vi "simulate-dashboard.vi"() -> ()   [LabVIEW 2019]
uses:
  <vilib>/Rock Robotics/WPI/ThirdParty/JAS_Junk/TrajLib/TypeDef/SWERVE_DRIVE_MODULE_POSITION.ctl
  <vilib>/Rock Robotics/WPI/ThirdParty/JAS_Junk/TrajLib/TypeDef/ROTATION2D.ctl
  <vilib>/Rock Robotics/WPI/ThirdParty/JAS_Junk/TrajLib/TypeDef/SWERVE_DRIVE_MODULE_STATE.ctl
  <vilib>/Rock Robotics/WPI/ThirdParty/JAS_Junk/TrajLib/TypeDef/CHASSIS_SPEEDS.ctl
  Swerve_Drive_System/SWERVE_DRIVE_GLOBALS.vi
  Simulation/SIMULATION_SIM_Globals.vi
  Sweve_Trajectory_Following/SWERVE_TRAJECTORY_GLOBALS.vi
  <vilib>/Rock Robotics/WPI/ThirdParty/JAS_Junk/TrajLib/Trajectory_Library.lvlib
panel:
  in  "Tab Control":T1(tab)
  out "Battery Voltage":dbl(graph)
  out "Swerve Motor Demands":T2(graph)
  out "Drive Motor Demands":T2(graph)
  out "Swerve Module Devices":T3(array[cluster])
  out "GyroReading_Degreees":dbl
  out "Encoder Distances":dbl[](array[numeric]) format="%17.2f"
  out "Encoder Velocities":dbl[](array[numeric]) format="%17.2f"
  out "Motor Demands":dbl[](array[numeric]) format="%17.2f"
  out "Battery Volts":dbl format="%16.2f"
  out "Swerve Module Positions":T4[](array[typedef]) {"Angle"."SIN" format="%13.4f"; "Angle"."COS" format="%13.4f"; "Angle"."VALUE" format="%13.4f"; "Distance" format="%19.2f"}
  out "Swerve Module States":T6[](array[typedef]) {"Angle"."SIN" format="%13.4f"; "Angle"."COS" format="%13.4f"; "Angle"."VALUE" format="%13.4f"; "Speed" format="%18.2f"}
  out "Adjusted Module State Demands":T6[](array[typedef]) {"Angle"."SIN" format="%13.4f"; "Angle"."COS" format="%13.4f"; "Angle"."VALUE" format="%13.4f"; "Speed" format="%20.2f"}
  out "Orientation Angle Dmd_Rad":dbl format="%17.3f"
  out "Drv Chassis Velocity DmD":T7 {"vOmega" format="%10.3f"; "vY" format="%10.3f"; "vX" format="%10.3f"}
  out "GyroHeading_Radians":dbl format="%17.2f"
  out "Orientation Angle Error_Rad":dbl format="%17.3f"
  out "Orientation Correct CO":dbl format="%17.3f"
  out "Adjusted Chassis Dmd":T7 {"vOmega" format="%10.3f"; "vY" format="%10.3f"; "vX" format="%10.3f"}
  out "Swerve Chassis Speed":T7 {"vOmega" format="%10.3f"; "vY" format="%10.3f"; "vX" format="%10.3f"}
  out "Mod Swerve in Deadband":bool
  out "Traj_OnTarget":bool
  # "SIMULATION"
  # "SWERVE DRIVE"
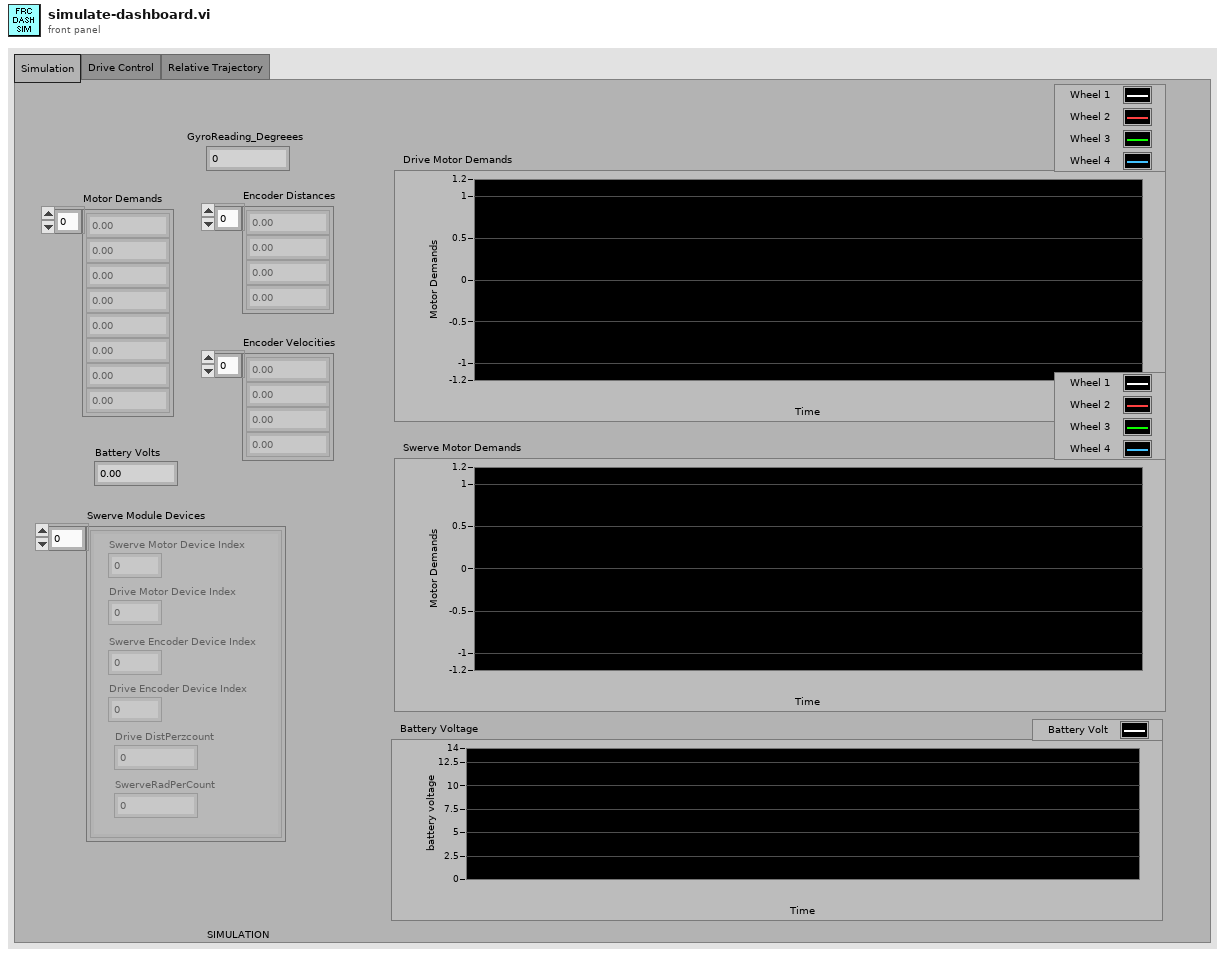
[diagram p1: front panel]
types:
  T1 = enum32{"Simulation", "Drive Control", "Relative Trajectory"}
  T2 = cluster{"Motor Dmd":dbl, "Motor Dmd":dbl, "Motor Dmd":dbl, "Motor Dmd":dbl}
  T3 = cluster{"Swerve Motor Device Index":i32, "Drive Motor Device Index":i32, "Swerve Encoder Device Index":i32, "Drive Encoder Device Index":i32, "Drive DistPerzcount":dbl, "SwerveRadPerCount":dbl}[]
  T4 = typedef "Trajectory_Library.lvlib/SWERVE_DRIVE_MODULE_POSITION.ctl" = cluster{"Distance":dbl, "Angle":T5, "P":bool}
  T5 = typedef "Trajectory_Library.lvlib/ROTATION2D.ctl" = cluster{"VALUE":dbl, "COS":dbl, "SIN":dbl}
  T6 = typedef "Trajectory_Library.lvlib/SWERVE_DRIVE_MODULE_STATE.ctl" = cluster{"Speed":dbl, "Angle":T5}
  T7 = typedef "Trajectory_Library.lvlib/CHASSIS_SPEEDS.ctl" = cluster{"vX":dbl, "vY":dbl, "vOmega":dbl}
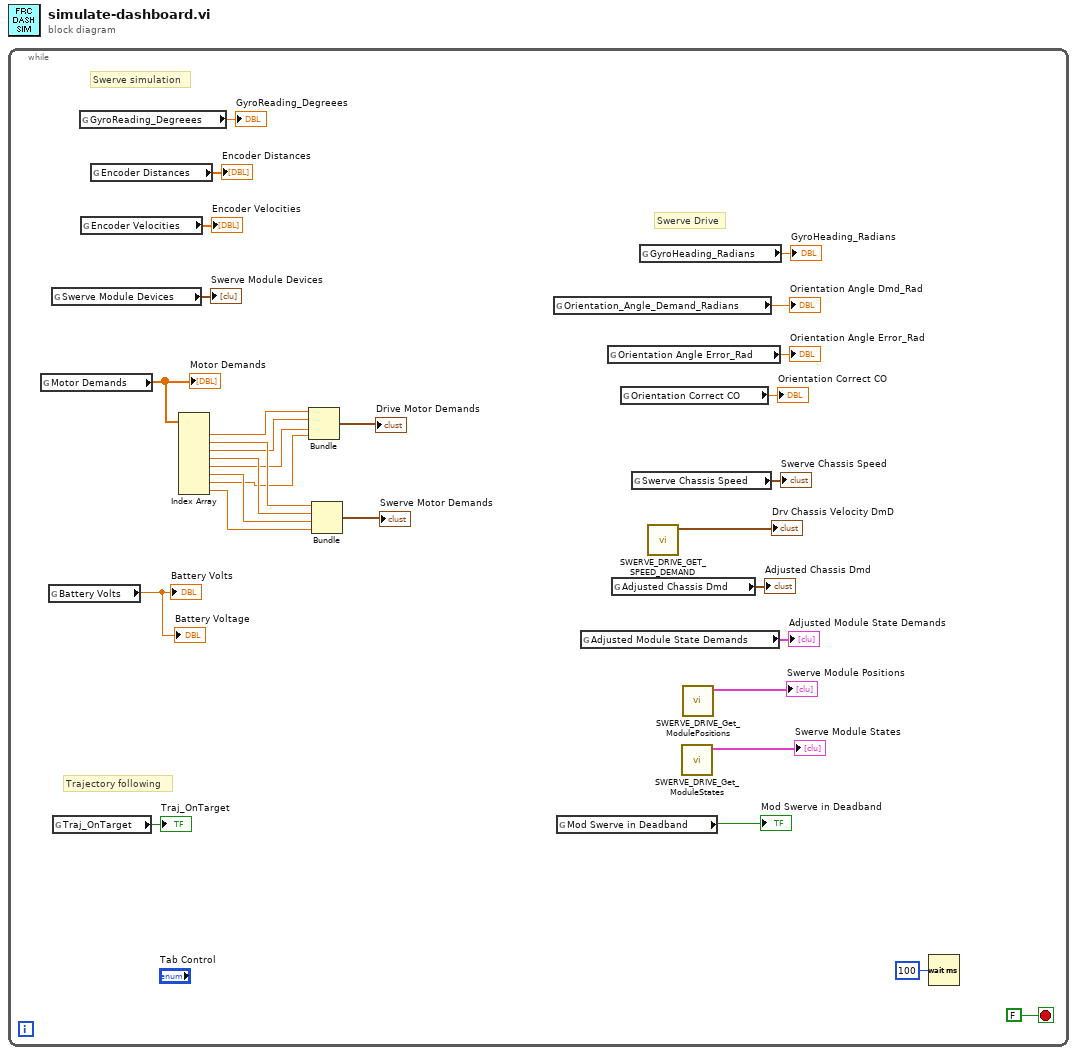
[diagram p0: block diagram]
diagram:
  n1 = while {
    stop <- FALSE stop-if-true
    # "Trajectory following"
    # "Swerve simulation"
    # "Swerve Drive"
    n2 = global read "SIMULATION_SIM_Globals.vi" "Motor Demands"() -> (w11:dbl[])
    "Motor Demands" <- w11
    n3 = global read "SIMULATION_SIM_Globals.vi" "Battery Volts"() -> (→"Battery Volts" →"Battery Voltage":dbl)
    n4 = global read "SIMULATION_SIM_Globals.vi" "Swerve Module Devices"() -> (→"Swerve Module Devices":T3)
    n5 = global read "SWERVE_TRAJECTORY_GLOBALS.vi" "Traj_OnTarget"() -> (→"Traj_OnTarget":bool)
    n6 = global read "SIMULATION_SIM_Globals.vi" "GyroReading_Degreees"() -> (→"GyroReading_Degreees":dbl)
    n7 = global read "SIMULATION_SIM_Globals.vi" "Encoder Velocities"() -> (→"Encoder Velocities":dbl[])
    n8 = global read "SIMULATION_SIM_Globals.vi" "Encoder Distances"() -> (→"Encoder Distances":dbl[])
    n9 = Index Array(array=w11) -> (element #1=w10:dbl, element #2=w9:dbl, element #3=w8:dbl, element #4=w7:dbl, element #5=w6:dbl, element #6=w5:dbl, element #7=w4:dbl, element #8=w3:dbl)  [unwired: 8 in]
    n10 = Bundle("Motor Dmd"=w10, "Motor Dmd"=w8, "Motor Dmd"=w6, "Motor Dmd"=w4) -> (→"Drive Motor Demands":T2)  [unwired: 1 in]
    n11 = Bundle("Motor Dmd"=w9, "Motor Dmd"=w7, "Motor Dmd"=w5, "Motor Dmd"=w3) -> (→"Swerve Motor Demands":T2)  [unwired: 1 in]
    n12 = global read "SWERVE_DRIVE_GLOBALS.vi" "Orientation_Angle_Demand_Radians"() -> (→"Orientation Angle Dmd_Rad":dbl)
    n13 = global read "SWERVE_DRIVE_GLOBALS.vi" "Mod Swerve in Deadband"() -> (→"Mod Swerve in Deadband":bool)
    n14 = global read "SWERVE_DRIVE_GLOBALS.vi" "Adjusted Module State Demands"() -> (→"Adjusted Module State Demands":T6[])
    n15 = global read "SWERVE_DRIVE_GLOBALS.vi" "Orientation Angle Error_Rad"() -> (→"Orientation Angle Error_Rad":dbl)
    n16 = global read "SWERVE_DRIVE_GLOBALS.vi" "Adjusted Chassis Dmd"() -> (→"Adjusted Chassis Dmd":T7)
    n17 = global read "SWERVE_DRIVE_GLOBALS.vi" "Orientation Correct CO"() -> (→"Orientation Correct CO":dbl)
    n18 = global read "SWERVE_DRIVE_GLOBALS.vi" "Swerve Chassis Speed"() -> (→"Swerve Chassis Speed":T7)
    n19 = global read "SWERVE_DRIVE_GLOBALS.vi" "GyroHeading_Radians"() -> (→"GyroHeading_Radians":dbl)
    n20 = call "SWERVE_DRIVE_GET_SPEED_DEMAND.vi"() -> ("Drv Chassis Velocity DmD"=→"Drv Chassis Velocity DmD":T7)  [unwired: 11 in]
    n21 = call "SWERVE_DRIVE_Get_ModuleStates.vi"() -> ("Swerve Module States"=→"Swerve Module States":T6[])  [unwired: 11 in]
    n22 = call "SWERVE_DRIVE_Get_ModulePositions.vi"() -> ("Swerve Module Positions"=→"Swerve Module Positions":T4[])  [unwired: 11 in]
    n23 = Wait (ms)(milliseconds to wait=u32 100) -> ()  [unwired: 1 out]
  }
